vi "test-linear-filter-noise-reduction-test-01B.vi"() -> (3 "Passed":bool)   [LabVIEW 2019]
uses:
  <vilib>/ptbypt/NI_PtbyPt.lvlib
  <vilib>/Rock Robotics/WPI/ThirdParty/JAS_Junk/TrajLib/Trajectory_Library.lvlib
panel:
  out "FilterError":dbl
  out "NoiseGenError":dbl
  out "Waveform Chart":cluster{"Output":dbl, "Output":dbl, dbl}(graph)
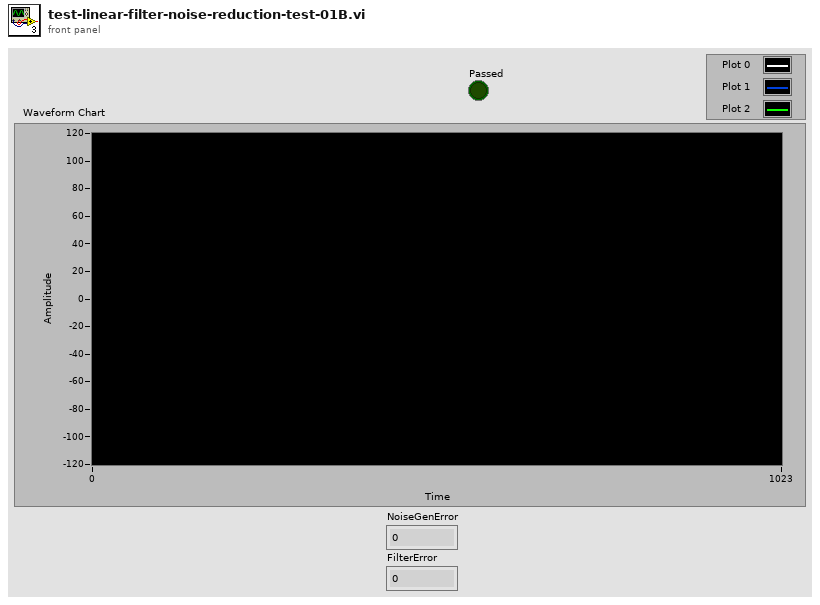
[diagram p1: front panel]
types:
  T1 = typedef "Trajectory_Library.lvlib/LINEAR_FILTER.ctl" = cluster{"InputGains":dbl[], "OutputGains":dbl[], "Inputs":dbl[], "Outputs":dbl[], "InGainCount":i32, "OutGainCount":i32}
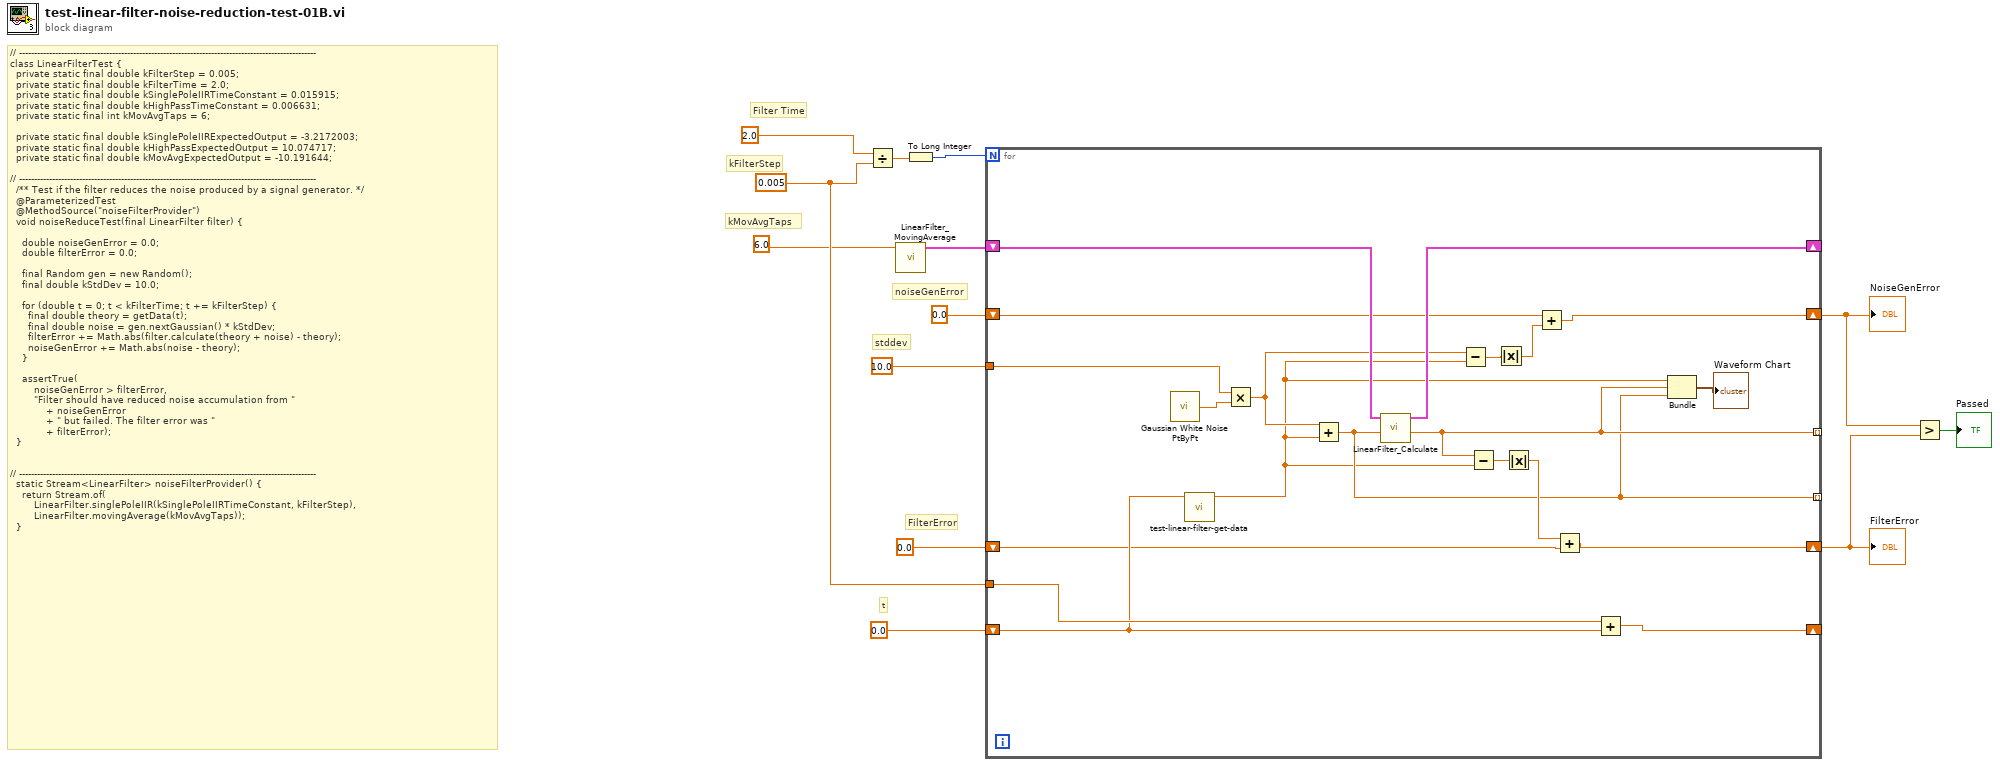
[diagram p0: block diagram]
diagram:
  w2 = 0.005
  # "kMovAvgTaps"
  # "stddev"
  # "t"
  # "kFilterStep"
  # "Filter Time"
  # "FilterError"
  # "noiseGenError"
  # "// ---------------------------------------------------------------------------------------------------\nclass LinearFilterTest {\n  private static final double kFilterStep = 0.005;\n  private static final double kFilterTime = 2.0;\n  private static final double kSinglePoleIIRTimeConstant = 0.015915;\n  private static final double kHighPassTimeConstant = 0.006631;\n  private static final int kMovAvgTaps = 6;\n\n  private static final double kSinglePoleIIRExpectedOutput = -3.2172003;\n  private static final double kHighPassExpectedOutput = 10.074717;\n  private static final double kMovAvgExpectedOutput = -10.191644;\n\n// ---------------------------------------------------------------------------------------------------\n  /** Test if the filter reduces the noise produced by a signal generator. */\n  @ParameterizedTest\n  @MethodSource(\"noiseFilterProvider\")\n  void noiseReduceTest(final LinearFilter filter) {\n\n    double noiseGenError = 0.0;\n    double filterError = 0.0;\n\n    final Random gen = new Random();\n    final double kStdDev = 10.0;\n\n    for (double t = 0; t < kFilterTime; t += kFilterStep) {\n      final double theory = getData(t);\n      final double noise = gen.nextGaussian() * kStdDev;\n      filterError += Math.abs(filter.calculate(theory + noise) - theory);\n      noiseGenError += Math.abs(noise - theory);\n    }\n\n    assertTrue(\n        noiseGenError > filterError,\n        \"Filter should have reduced noise accumulation from \"\n            + noiseGenError\n            + \" but failed. The filter error was \"\n            + filterError);\n  }\n\n\n// ---------------------------------------------------------------------------------------------------\n  static Stream<LinearFilter> noiseFilterProvider() {\n    return Stream.of(\n        LinearFilter.singlePoleIIR(kSinglePoleIIRTimeConstant, kFilterStep),\n        LinearFilter.movingAverage(kMovAvgTaps));\n  }"
  n1 = Divide(x=2.0, y=w2) -> (x/y=w13:dbl)
  n2 = call <vilib>:"LinearFilter_MovingAverage.vi"("Samples"=6.0 ("TimeConstant")) -> ("LINEAR_FILTER"=w3:T1)  [unwired: 9 in, 1 out]
  n3 = To Long Integer(number=w13) -> (32bit integer=w12:i32)
  n4 = for {
    N: w12 -> [_]
    shift-right: [w32] -> _
    shift-left: 0.0 -> [w31]
    tunnel: w2 -> [w33]
    tunnel: 10.0 -> [w29]
    shift-right: [w27] -> _
    shift-left: w3 -> [w28]
    tunnel: [w15] -> _ mode=indexing
    tunnel: [w16] -> _ mode=indexing
    shift-right: [w24] -> w5
    shift-left: 0.0 -> [w23]
    shift-right: [w20] -> w6
    shift-left: 0.0 -> [w19]
    n5 = call <vilib>:"Gaussian White Noise PtByPt.vi"() -> ("Gaussian white noise"=w30:dbl)  [unwired: 3 in]
    n6 = call "test-linear-filter-get-data.vi"("T"=w31) -> ("Output"=w14:dbl)  [unwired: 10 in]
    n7 = Multiply(x=w29, y=w30) -> (x*y=w22:dbl)
    n8 = Add(x=w22, y=w14) -> (x+y=w15:dbl)
    n9 = call <vilib>:"LinearFilter_Calculate.vi"("Input"=w15, "In LINEAR_FILTER"=w28) -> ("Output"=w16:dbl, "Out LINEAR_FILTER"=w27:T1)  [unwired: 8 in]
    n10 = Subtract(x=w22, y=w14) -> (x-y=w21:dbl)
    n11 = Subtract(x=w16, y=w14) -> (x-y=w26:dbl)
    n12 = Absolute Value(x=w21) -> (abs(x)=w18:dbl)
    n13 = Absolute Value(x=w26) -> (abs(x)=w25:dbl)
    n14 = Add(x=w19, y=w18) -> (x+y=w20:dbl)
    n15 = Add(x=w25, y=w23) -> (x+y=w24:dbl)
    n16 = Add(x=w33, y=w31) -> (x+y=w32:dbl)
    n17 = Bundle("Output"=w14, "Output"=w16, w15) -> (→"Waveform Chart":cluster{"Output":dbl, "Output":dbl, dbl})  [unwired: 1 in]
  }
  "NoiseGenError" <- w6
  "FilterError" <- w5
  n18 = Greater?(x=w6, y=w5) -> (0:→"Passed":bool)
